vi "WPI_DashboardNTL FF to New Position2.vi"(7 "Version":i32=1, 8 "VI Refnum":refnum<vi>, 10 "TimeOffset (s)":dbl, 11 "Byte Stream File in":refnum<file>) -> (0 "Strings":T1, 1 "Unchanged":bool, 2 "New time (s)":dbl, 3 "Byte Stream File out":refnum<file>)   [LabVIEW 2017]
uses:
  <vilib>/Rock Robotics/WPI/Dashboard/WPI_DashboardLoggingRecord.ctl
  <vilib>/Rock Robotics/Network Tables/Protocol Operations.ctl
  <vilib>/Rock Robotics/Network Tables/Field Data.ctl
  <vilib>/Rock Robotics/Network Tables/Field Type.ctl
  <vilib>/Rock Robotics/Network Tables/Sequence.ctl
  <vilib>/Rock Robotics/WPI/Dashboard/WPI_DashboardLogging Global.vi
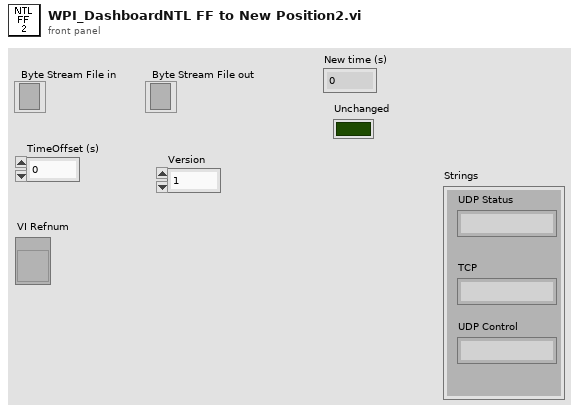
[diagram p1: front panel]
types:
  T1 = cluster{"UDP Status":string, "TCP":string, "UDP Control":string}
  T2 = typedef "Protocol Operations.ctl" = enum16{"Unknown", "Keep Alive", "Client Hello", "Version not supported", "Server Hello Complete", "Assign", "Update", "No Op", "Server Hello", "Client Hello Complete", "Update Flags", "Delete Entry", "Delete All", "RPC Exec", "RPC Response"}
  T3 = typedef "Field Data.ctl" = cluster{"Dbl":dbl, "String":string, "Type":T4, "Boolean":bool, "Sequence #":T5, "Flags":u8}
  T4 = typedef "Field Type.ctl" = enum8{"Invalid", "Bool", "Numeric", "String", "Raw", "Boolean Array", "Numeric Array", "String Array", "RPC"}
  T5 = typedef "Sequence.ctl" = u16
  T6 = cluster{"time Ofst":i32, "video index":i32, "UDP Status":string, "TCP":string, "UDP Control":string, "NT Updates":cluster{"Operation":T2, "Name":string, "Field Value":T3}[]}
  T7 = typedef "WPI_DashboardLoggingRecord.ctl" = cluster{"time Ofst":i32, "video index":i32, "video index 2":i32, "video index 3":i32, "video index 4":i32, "UDP Status":string, "TCP":string, "UDP Control":string, "NT Updates":cluster{"Operation":T2, "Name":string, "Field Value":T3}[]}
  T8 = cluster{"Operation":T2, "Name":string, "Field Value":T3}[]
  T9 = cluster{"video index":i32, "video index 2":i32, "video index 3":i32, "video index 4":i32}
  T10 = cluster{"Video 1":i32, "Video 2":i32, "Video 3":i32, "Video 4":i32}
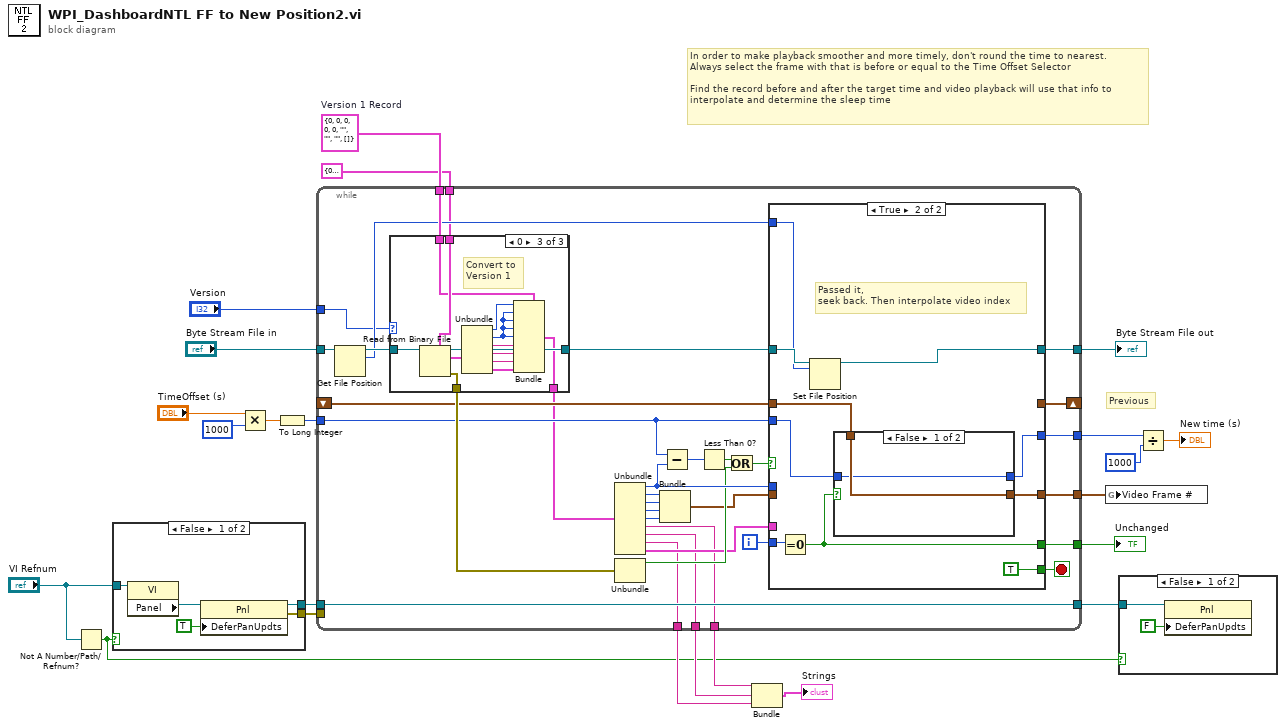
[diagram p0: block diagram]
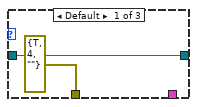
[diagram p4: hidden frame]
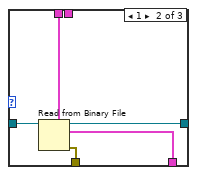
[diagram p5: hidden frame]
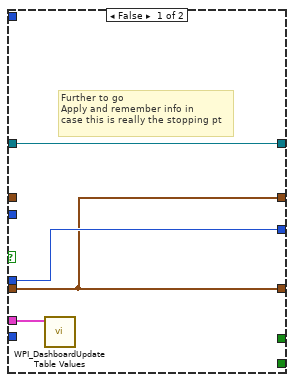
[diagram p6: hidden frame]
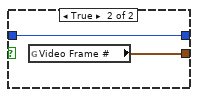
[diagram p7: hidden frame]
diagram:
  w5 = T7 {"time Ofst"=0, "video index"=0, "video index 2"=0, "video index 3"=0, "video index 4"=0, "UDP Status"="", "TCP"="", "UDP Control"="", "NT Updates"=[]}  # Version 1 Record
  # "Previous"
  # "In order to make playback smoother and more timely, don't round the time to nearest.\nAlways select the frame with that is before or equal to the Time Offset Selector\n\nFind the record before and after the target time and video playback will use that info to\ninterpolate and determine the sleep time"
  n1 = Not A Number/Path/Refnum?(number/path/refnum="VI Refnum") -> (NaN/Path/Refnum?=w1:bool)
  n2 = case shown="False" w1 {
    tunnel: [w26 _] -> w11
    tunnel: [w25 _] -> w10
    tunnel: "VI Refnum" -> [w24 _]
    frame False {
      n3 = property class="VI"(reference=w24) -> ("Panel"=w28:refnum<vi>)  [unwired: 1 in, 2 out]
      n4 = property class="Pnl"(reference=w28, "DeferPanUpdts"=TRUE ("Defer Panel Updates")) -> (reference out=w26:refnum<vi>, error out=w25:errorcluster)  [unwired: 1 in]
    }
    frame True {
    }
  }
  n5 = Multiply(x="TimeOffset (s)", y=1000) -> (x*y=w18:dbl)
  n6 = To Long Integer(number=w18) -> (32bit integer=w17:i32)
  n7 = while {
    tunnel: w5 -> [w61]
    tunnel: "Byte Stream File in" -> [w48]
    tunnel: [w58] -> w22
    tunnel: w17 -> [w54]
    shift-right: [w57] -> _
    shift-left: _ -> [w56]
    tunnel: [w52] -> w21
    tunnel: [w50] -> w14
    tunnel: [w49] -> w13
    tunnel: [w36] -> w9
    tunnel: [w38] -> w8
    tunnel: w11 -> [w40]
    tunnel: [w40] -> w12
    tunnel: w10 -> [_]
    tunnel: [w37] -> w7
    tunnel: "Version" -> [w30]
    tunnel: T6 {"time Ofst"=0, "video index"=0, "UDP Status"="", "TCP"="", "UDP Control"="", "NT Updates"=[]} ("output cluster") -> [w29]
    i -> [w51]
    stop <- w41 stop-if-true
    n8 = Get File Position(7:w48) -> (2:w46:i64, 3:w47:refnum<file>)  [unwired: 1 in, 1 out]
    n9 = case shown="0" w30 {
      tunnel: w61 -> [_ w68 w76]
      tunnel: [errorcluster {"status"=TRUE, "code"=4, "source"=""} ("error constant") w67 w81] -> w60
      tunnel: [w62 w66 w80] -> w59
      tunnel: [_ w65 w69] -> w53
      tunnel: w47 -> [w62 w64 w79]
      tunnel: w29 -> [_ _ w78]
      frame Default {
      }
      frame 1 {
        n10 = Read from Binary File(5:w68, 11:w64) -> (0:w67:errorcluster, 2:w65:T7, 3:w66:refnum<file>)  [unwired: 4 in, 1 out]
      }
      frame 0 {
        # "Convert to\nVersion 1"
        n11 = Read from Binary File(5:w78, 11:w79) -> (0:w81:errorcluster, 2:w77:T6, 3:w80:refnum<file>)  [unwired: 4 in, 1 out]
        n12 = Unbundle(w77) -> ("time Ofst"=w71:i32, "video index"=w70:i32, "UDP Status"=w72:string, "TCP"=w73:string, "UDP Control"=w74:string, "NT Updates"=w75:T8)
        n13 = Bundle(cluster=w76, "time Ofst"=w71, "video index"=w70, "video index 2"=w70, "video index 3"=w70, "video index 4"=w70, "UDP Status"=w72, "TCP"=w73, "UDP Control"=w74, "NT Updates"=w75) -> (w69:T7)
      }
    }
    n14 = Unbundle(w53) -> ("time Ofst"=w55:i32, "video index"=w35:i32, "video index 2"=w34:i32, "video index 3"=w33:i32, "video index 4"=w32:i32, "UDP Status"=w36:string, "TCP"=w37:string, "UDP Control"=w38:string, "NT Updates"=w39:T8)
    n15 = Unbundle(w60) -> ("status"=w42:bool)  [unwired: 2 out]
    n16 = Bundle("video index"=w35, "video index 2"=w34, "video index 3"=w33, "video index 4"=w32) -> (w31:T9)  [unwired: 1 in]
    n17 = Subtract(x=w54, y=w55) -> (x-y=w43:i32)
    n18 = Less Than 0?(x=w43) -> (x < 0?=w45:bool)
    n19 = Or(x=w45, y=w42) -> (x .or. y?=w44:bool)
    n20 = case shown="True" w44 {
      tunnel: w59 -> [w84 w94]
      tunnel: [w84 w93] -> w58
      tunnel: [w82 _] -> w57
      tunnel: w56 -> [_ w86]
      tunnel: [_ TRUE] -> w41
      tunnel: w55 -> [w85 _]
      tunnel: w54 -> [_ w87]
      tunnel: w39 -> [w83 _]
      tunnel: [w85 w89] -> w52
      tunnel: w51 -> [_ w92]
      tunnel: [_ w88] -> w50
      tunnel: w31 -> [w82 _]
      tunnel: [w82 w90] -> w49
      tunnel: w46 -> [_ w91]
      frame False {
        # "Further to go\nApply and remember info in\ncase this is really the stopping pt"
        n21 = call <vilib>:"WPI_DashboardUpdate Table Values.vi"("Data Values"=w83) -> ()  [unwired: 11 in]
      }
      frame True {
        # "Passed it,\nseek back. Then interpolate video index"
        n22 = Equal To 0?(x=w92) -> (x = 0?=w88:bool)
        n23 = Set File Position(offset (in bytes) (0)=w91, refnum=w94) -> (refnum out=w93:refnum<file>)  [unwired: 2 in, 1 out]
        n24 = case shown="False" w88 {
          tunnel: [w97 w98] -> w90
          tunnel: w86 -> [w97 _]
          tunnel: [w96 w99] -> w89
          tunnel: w87 -> [w96 w99]
          frame False {
          }
          frame True {
            n25 = global read "WPI_DashboardLogging Global.vi" "Video Frame #"() -> (w98:T10)
          }
        }
      }
    }
  }
  "Byte Stream File out" <- w22
  "Unchanged" <- w14
  n26 = Bundle("UDP Status"=w9, "TCP"=w7, "UDP Control"=w8) -> (→"Strings":T1)  [unwired: 1 in]
  n27 = global write "WPI_DashboardLogging Global.vi" "Video Frame #"(w13) -> ()
  n28 = case shown="False" w1 {
    tunnel: w12 -> [w100 _]
    frame False {
      n29 = property class="Pnl"(reference=w100, "DeferPanUpdts"=FALSE ("Defer Panel Updates")) -> ()  [unwired: 1 in, 2 out]
    }
    frame True {
    }
  }
  n30 = Divide(x=w21, y=1000) -> (x/y=→"New time (s)":dbl)
